vi "Create from SFTP Directory.vi"(8 "Error In":errorcluster, 11 "SFTP Directory In":refnum<class "SFTP Directory.lvclass">) -> (0 "Error Out":errorcluster, 2 "SFTP Attributes":refnum<class "SFTP Attributes.lvclass">, 3 "SFTP Directory Out":refnum<class "SFTP Directory.lvclass">)   [LabVIEW 2021, in "Field_RnD_Services_LIBSSH2_Toolkit.lvlib" / "SFTP Attributes.lvclass"]
doc: "Passes through the SFTP Directory object but obtains the SSH context for the SFTP Directory object to create a new SFTP Attributes object."
uses:
  SFTP Attributes.lvclass
  SFTP Directory/SFTP Directory.lvclass
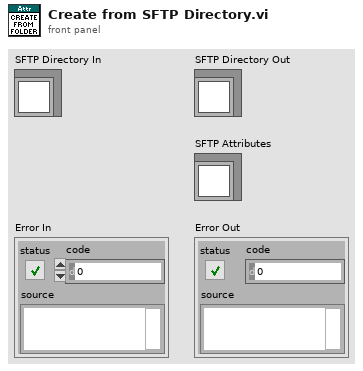
[diagram p1: front panel]
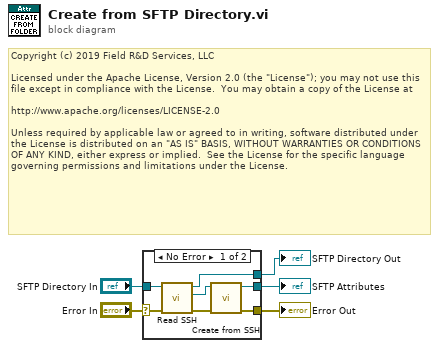
[diagram p0: block diagram]
diagram:
  # "Copyright (c) 2019 Field R&D Services, LLC\n\nLicensed under the Apache License, Version 2.0 (the \"License\"); you may not use this file except in compliance with the License.  You may obtain a copy of the License at\n\nhttp://www.apache.org/licenses/LICENSE-2.0\n\nUnless required by applicable law or agreed to in writing, software distributed under the License is distributed on an \"AS IS\" BASIS, WITHOUT WARRANTIES OR CONDITIONS OF ANY KIND, either express or implied.  See the License for the specific language governing permissions and limitations under the License."
  n1 = case shown="No Error" "Error In" {
    selector: "Error In" -> [w7 w14]
    tunnel: [w11 w14] -> w4
    tunnel: [w12 _] -> w3
    tunnel: "SFTP Directory In" -> [w10 w13]
    tunnel: [w6 w13] -> w1
    frame No Error {
      n2 = call "Read SSH.vi"("Error In"=w7, "SFTP Directory In"=w10) -> ("Error Out"=w8:errorcluster, "SSH"=w9:refnum<class "SSH.lvclass">, "SFTP Directory Out"=w6:refnum<class "SFTP Directory.lvclass">)  [unwired: 7 in]
      n3 = call "Create from SSH.vi"("Error In"=w8, "SSH"=w9) -> ("Error Out"=w11:errorcluster, "SFTP Attributes"=w12:refnum<class "SFTP Attributes.lvclass">)  [unwired: 8 in]
    }
    frame Error {
    }
  }
  "Error Out" <- w4
  "SFTP Attributes" <- w3
  "SFTP Directory Out" <- w1
